vi "Builtins.vi"(6 "args":string[](array[string]), 7 "QD Plugins Dir":path, 8 "error in (no error)":errorcluster, 9 "Shift?":bool, 10 "Focus":enum8{"FP", "BD"}(ring), 11 "VI Refnum":refnum<vi>) -> (0 "error out":errorcluster)   [LabVIEW 2019]
doc: "Built-in script shortcuts\n\nUsage: Ctrl-Space + \"<shortcut>\" + Ctrl-S\n\nCreated by: Ryan Pacini\n\n[SCRIPT]\n--=Rename Label\n--c=Rename Caption\n--iconlib=Edit Library Icon\n0=Open in File Explore\na=Arrange\naa=Align Left Edges\nad=Align Right Edges\nah=Align Horizontal Centers\nas=Align Bottom Edges\nav=Align Vertical Centers\naw=Align Top Edges\nc=Connect Pane\ncf=Cluster Size Fit\nch=Cluster Size Horizontally\ncn=Cluster Size None\ncv=Cluster Size Vertically\nd=Distribute Vertical Compress\nda=Distribute Left Edges\ndd=Distribute Right Edges\ndf=Distribute Horizontal Compress \ndh=Distribute Horizontal Centers\ndhg=Distribute Horizontal Gap\nds=Distribute Bottom Edges\ndv=Distribute Vertical Centers\ndvg=Distribute Vertical Gap\ndw=Distribute Top Edges\ne=Resizes Window\ner=Error Structure\nhb=Hide Inc/Dec Buttons\nhc=Hide Caption\nhi=Hide Index Display\nhl=Hide Label\nhr=Hide Radix\nhs=Hide Scrollbars\nm=Merge Icon Layers\no=Reset Panel Origins\nrb=Radix Binary or Backslash\nrd=Radix Decimal or Normal\nrx=Radix Hex\nsb=Show Inc/Dec Buttons\nsc=Show Caption\nsi=Show Index Display\nsl=Show Label\nss=Show Scrollbars\nsel=Select Controls and Indicators\nselc=Select Controls\nseli=Select Indicators\nseln=Select None\nsg=Snap to Panel Grid\nu8=Change to U8\nu16=Change to U16\nu32=Change to U32\nu64=Change to U64\ni8=Change to I8\ni16=Change to I16\ni32=Change to I32\ni64=Change to I64\nsgl=Change to SGL\ndbl=Change to DBL\next=Change to EXT\ncsg=Change to CSG\ncdb=Change to CDB\ncxt=Change to CXT\nvi=VI Voodoo"
uses:
  _Builtins/Align.ctl
  <vilib>/numeric/LVNumericRepresentation.ctl
  _Builtins/Distribute.ctl
  _Builtins/Selection.ctl
  _Builtins/Builtins.lvlib
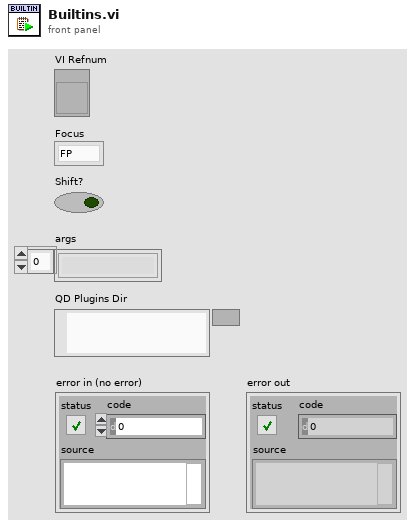
[diagram p1: front panel]
types:
  T1 = typedef "Builtins.lvlib/Align.ctl" = enum8{"Top Edges", "Vertical Centers", "Bottom Edges", "Left Edges", "Horizontal Centers", "Right Edges"}
  T2 = typedef "LVNumericRepresentation.ctl" = enum32{"Extended Precision", "Double Precision", "Single Precision", "Long", "Word", "Byte", "Unsigned Long", "Unsigned Word", "Unsigned Byte", "Complex Extended", "Complex Double", "Complex Single", "Quad", "Unsigned Quad", "Fixed-Point"}
  T3 = enum8{"None", "SizeToFit", "Horizontally", "Vertically"}
  T4 = typedef "Builtins.lvlib/Distribute.ctl" = enum8{"Top Edges", "Vertical Centers", "Bottom Edges", "Vertical Gap", "Vertical Compress", "Left Edges", "Horizontal Centers", "Right Edges", "Horizontal Gap", "Horizontal Compress"}
  T5 = typedef "Builtins.lvlib/Selection.ctl" = enum8{"None", "Controls", "Indicators", "Both"}
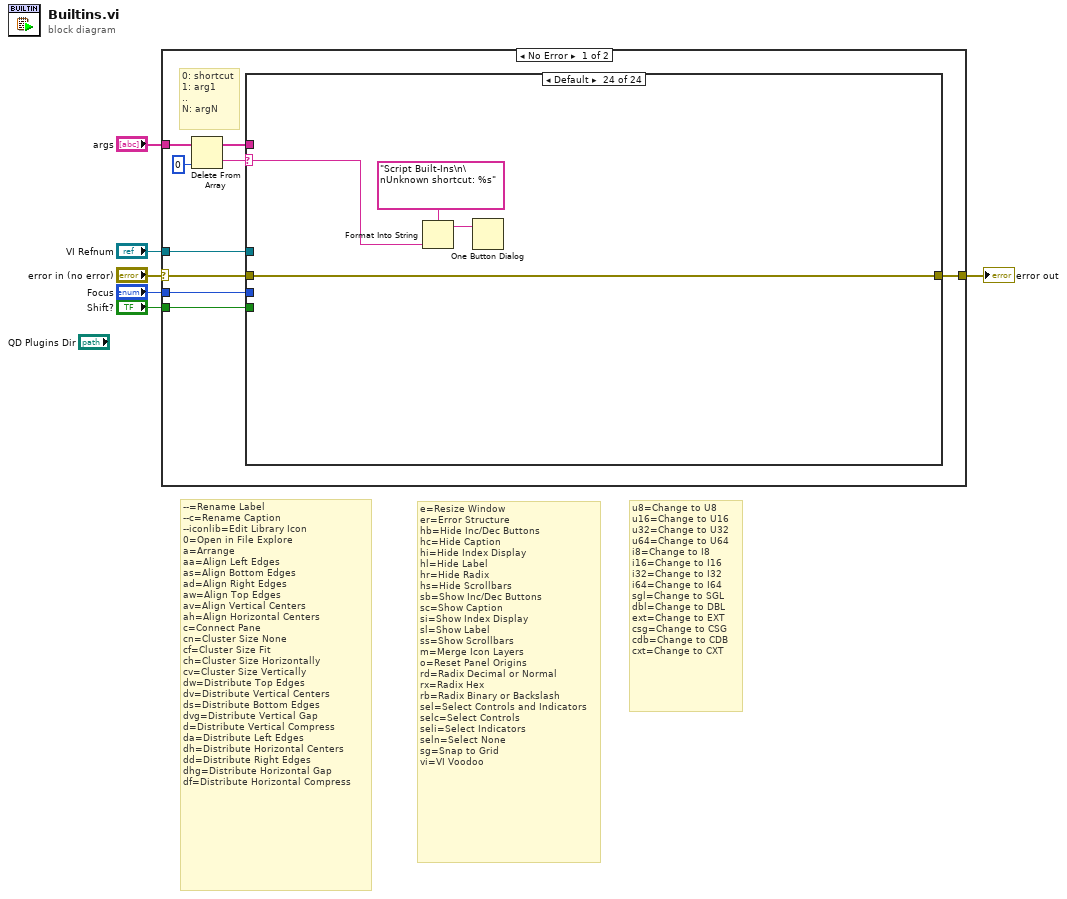
[diagram p0: block diagram]
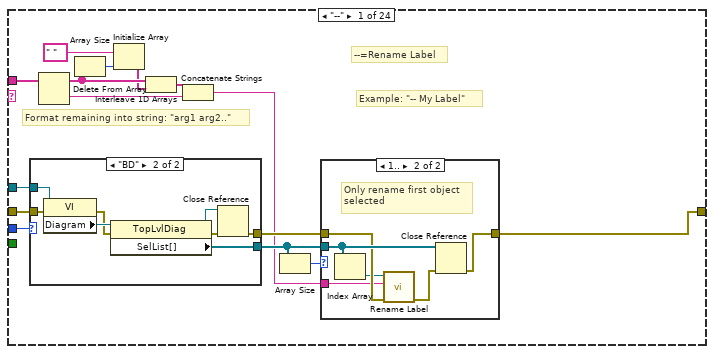
[diagram p2: hidden frame]
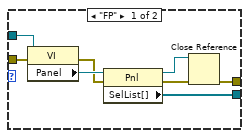
[diagram p3: hidden frame]
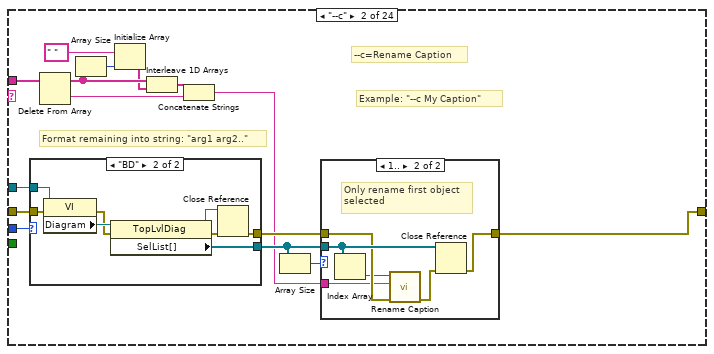
[diagram p5: hidden frame]
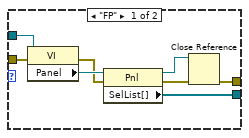
[diagram p6: hidden frame]
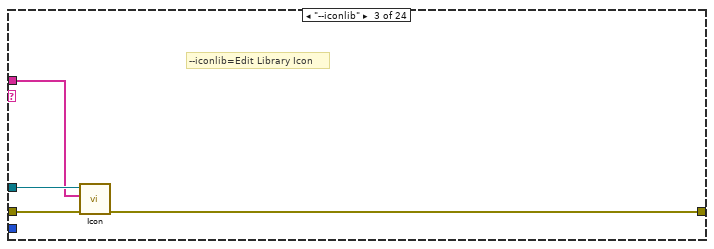
[diagram p8: hidden frame]
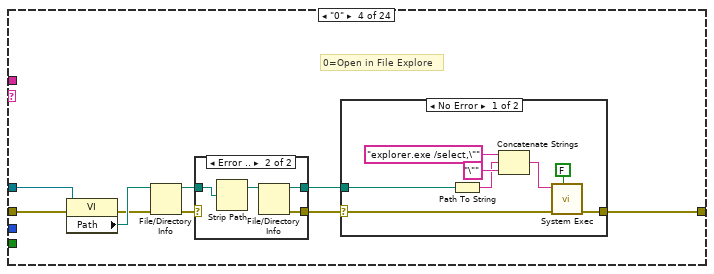
[diagram p9: hidden frame]
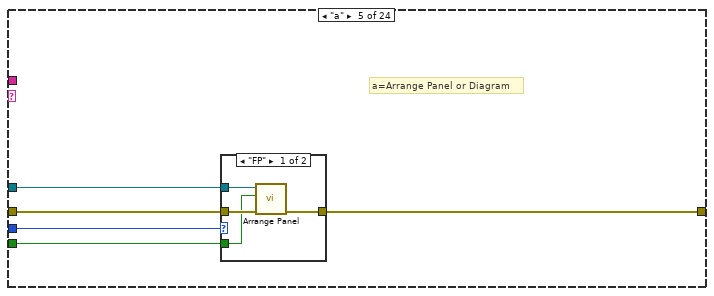
[diagram p12: hidden frame]
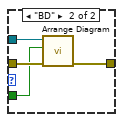
[diagram p13: hidden frame]
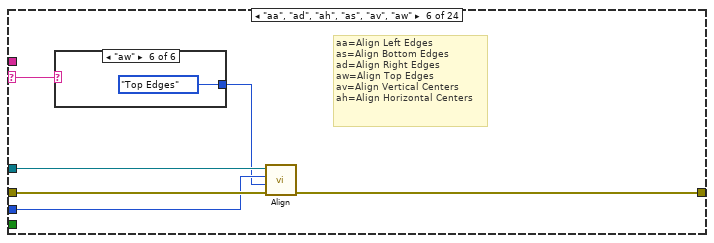
[diagram p14: hidden frame]
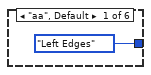
[diagram p15: hidden frame]
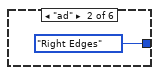
[diagram p16: hidden frame]
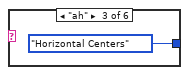
[diagram p17: hidden frame]
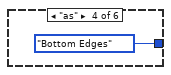
[diagram p18: hidden frame]
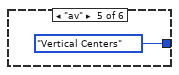
[diagram p19: hidden frame]
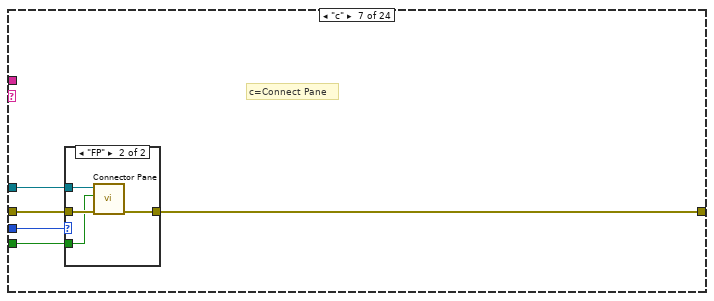
[diagram p20: hidden frame]
diagram:
  # "u8=Change to U8\nu16=Change to U16\nu32=Change to U32\nu64=Change to U64\ni8=Change to I8\ni16=Change to I16\ni32=Change to I32\ni64=Change to I64\nsgl=Change to SGL\ndbl=Change to DBL\next=Change to EXT\ncsg=Change to CSG\ncdb=Change to CDB\ncxt=Change to CXT"
  # "e=Resize Window\ner=Error Structure\nhb=Hide Inc/Dec Buttons\nhc=Hide Caption\nhi=Hide Index Display\nhl=Hide Label\nhr=Hide Radix\nhs=Hide Scrollbars\nsb=Show Inc/Dec Buttons\nsc=Show Caption\nsi=Show Index Display\nsl=Show Label\nss=Show Scrollbars\nm=Merge Icon Layers\no=Reset Panel Origins\nrd=Radix Decimal or Normal\nrx=Radix Hex\nrb=Radix Binary or Backslash\nsel=Select Controls and Indicators\nselc=Select Controls\nseli=Select Indicators\nseln=Select None\nsg=Snap to Grid\nvi=VI Voodoo"
  # "--=Rename Label\n--c=Rename Caption\n--iconlib=Edit Library Icon\n0=Open in File Explore\na=Arrange\naa=Align Left Edges\nas=Align Bottom Edges\nad=Align Right Edges\naw=Align Top Edges\nav=Align Vertical Centers\nah=Align Horizontal Centers\nc=Connect Pane\ncn=Cluster Size None\ncf=Cluster Size Fit\nch=Cluster Size Horizontally\ncv=Cluster Size Vertically\ndw=Distribute Top Edges\ndv=Distribute Vertical Centers\nds=Distribute Bottom Edges\ndvg=Distribute Vertical Gap\nd=Distribute Vertical Compress\nda=Distribute Left Edges\ndh=Distribute Horizontal Centers\ndd=Distribute Right Edges\ndhg=Distribute Horizontal Gap\ndf=Distribute Horizontal Compress"
  n1 = case shown="No Error" "error in (no error)" {
    selector: "error in (no error)" -> [w15 w387]
    tunnel: "VI Refnum" -> [w14 _]
    tunnel: "Focus" -> [w13 _]
    tunnel: "Shift?" -> [w11 _]
    tunnel: "args" -> [w10 _]
    tunnel: [w12 w387] -> w1
    frame No Error {
      # "0: shortcut\n1: arg1\n..\nN: argN"
      n2 = Delete From Array(array=w10, index=0) -> (deleted portion=w9:string, array with subset deleted=w8:string[])  [unwired: 1 in]
      n3 = case shown="Default" w9 {
        selector: w9 -> [_ _ _ _ _ w133 _ w159 w213 w223 _ _ w253 w267 w282 w296 w310 w323 _ _ w345 _ _ w385]
        tunnel: w15 -> [w30 w68 w95 w104 w124 w138 w149 w158 w212 w228 w241 w246 w252 w266 w280 w294 w308 w322 w334 w338 w349 w357 w378 w386]
        tunnel: w14 -> [w29 w67 w94 w103 w123 w137 w148 w157 w211 w227 w242 w245 w251 w265 w279 w293 w307 w321 w335 w339 w348 w356 w377 _]
        tunnel: w13 -> [w24 w62 _ _ w121 w135 w146 w155 w210 w226 w239 w243 w250 w264 w278 w292 w306 w320 _ w336 w346 w354 w372 _]
        tunnel: [w27 w65 w93 w102 w122 w136 w147 w156 w207 w225 w240 w244 w247 w261 w276 w289 w303 w317 w333 w337 w347 w355 w367 w386] -> w12
        tunnel: w11 -> [_ _ _ _ w120 _ w145 _ _ _ _ _ _ _ _ _ _ _ _ _ _ _ _ _]
        tunnel: w8 -> [w17 w55 w92 _ _ _ _ _ _ _ _ _ _ _ _ _ _ _ _ _ _ _ _ _]
        frame "--" {
          # "Example: \"-- My Label\""
          # "Format remaining into string: \"arg1 arg2..\""
          # "--=Rename Label"
          n4 = case shown="\"BD\"" w24 {
            tunnel: w30 -> [w38 w46]
            tunnel: w29 -> [w37 w45]
            tunnel: [w33 w41] -> w28
            tunnel: [w31 w39] -> w25
            frame "FP" {
              n5 = property class="VI"(reference=w37, error in=w38) -> (error out=w35:errorcluster, "Panel"=w36:refnum<vi>)  [unwired: 1 out]
              n6 = property class="Pnl"(reference=w36, error in=w35) -> (reference out=w34:refnum<vi>, error out=w32:errorcluster, "SelList[]"=w33:refnum<vi>[])
              n7 = Close Reference(reference=w34, error in (no error)=w32) -> (error out=w31:errorcluster)
            }
            frame "BD" {
              n8 = property class="VI"(reference=w45, error in=w46) -> (error out=w43:errorcluster, "Diagram"=w44:refnum<vi>)  [unwired: 1 out]
              n9 = property class="TopLvlDiag"(reference=w44, error in=w43) -> (reference out=w42:refnum<vi>, error out=w40:errorcluster, "SelList[]"=w41:refnum<vi>[])
              n10 = Close Reference(reference=w42, error in (no error)=w40) -> (error out=w39:errorcluster)
            }
          }
          n11 = Delete From Array(array=w17) -> (deleted portion=w18:string, array with subset deleted=w20:string[])  [unwired: 2 in]
          n12 = Array Size(array=w20) -> (size(s)=w22:i32)
          n13 = Initialize Array(" ", w22) -> (w19:string[])
          n14 = Interleave 1D Arrays(w20, w19) -> (w23:string[])
          n15 = Concatenate Strings(w23, w18) -> (w16:string)
          n16 = Array Size(array=w28) -> (size(s)=w26:i32)
          n17 = case shown="1.." w26 {
            tunnel: w25 -> [w47 w51]
            tunnel: w28 -> [_ w53]
            tunnel: w16 -> [_ w48]
            tunnel: [w47 w52] -> w27
            frame ..0 {
              # "Nothing selected"
            }
            frame 1.. {
              # "Only rename first object\nselected"
              n18 = Index Array(array=w53) -> (element=w50:refnum<vi>)  [unwired: 1 in]
              n19 = call "Rename Label.vi"("error in (no error)"=w51, "Label"=w48, "GObject in"=w50) -> ("error out"=w49:errorcluster)  [unwired: 6 in, 2 out]
              n20 = Close Reference(reference=w53, error in (no error)=w49) -> (error out=w52:errorcluster)
            }
          }
        }
        frame "--c" {
          # "Example: \"--c My Caption\""
          # "Format remaining into string: \"arg1 arg2..\""
          # "--c=Rename Caption"
          n21 = case shown="\"BD\"" w62 {
            tunnel: w68 -> [w76 w84]
            tunnel: w67 -> [w75 w83]
            tunnel: [w71 w79] -> w66
            tunnel: [w69 w77] -> w63
            frame "FP" {
              n22 = property class="VI"(reference=w75, error in=w76) -> (error out=w73:errorcluster, "Panel"=w74:refnum<vi>)  [unwired: 1 out]
              n23 = property class="Pnl"(reference=w74, error in=w73) -> (reference out=w72:refnum<vi>, error out=w70:errorcluster, "SelList[]"=w71:refnum<vi>[])
              n24 = Close Reference(reference=w72, error in (no error)=w70) -> (error out=w69:errorcluster)
            }
            frame "BD" {
              n25 = property class="VI"(reference=w83, error in=w84) -> (error out=w81:errorcluster, "Diagram"=w82:refnum<vi>)  [unwired: 1 out]
              n26 = property class="TopLvlDiag"(reference=w82, error in=w81) -> (reference out=w80:refnum<vi>, error out=w78:errorcluster, "SelList[]"=w79:refnum<vi>[])
              n27 = Close Reference(reference=w80, error in (no error)=w78) -> (error out=w77:errorcluster)
            }
          }
          n28 = Delete From Array(array=w55) -> (deleted portion=w56:string, array with subset deleted=w58:string[])  [unwired: 2 in]
          n29 = Array Size(array=w58) -> (size(s)=w60:i32)
          n30 = Initialize Array(" ", w60) -> (w57:string[])
          n31 = Interleave 1D Arrays(w58, w57) -> (w61:string[])
          n32 = Concatenate Strings(w61, w56) -> (w54:string)
          n33 = Array Size(array=w66) -> (size(s)=w64:i32)
          n34 = case shown="1.." w64 {
            tunnel: w63 -> [w85 w89]
            tunnel: w66 -> [_ w91]
            tunnel: w54 -> [_ w87]
            tunnel: [w85 w90] -> w65
            frame ..0 {
              # "Nothing selected"
            }
            frame 1.. {
              # "Only rename first object\nselected"
              n35 = Index Array(array=w91) -> (element=w88:refnum<vi>)  [unwired: 1 in]
              n36 = call "Rename Caption.vi"("error in (no error)"=w89, "Caption"=w87, "GObject in"=w88) -> ("error out"=w86:errorcluster)  [unwired: 6 in, 2 out]
              n37 = Close Reference(reference=w91, error in (no error)=w86) -> (error out=w90:errorcluster)
            }
          }
        }
        frame "--iconlib" {
          # "--iconlib=Edit Library Icon"
          n38 = call "Icon.vi"("error in (no error)"=w95, "Args"=w92, "VI Refnum in"=w94) -> ("error out"=w93:errorcluster)  [unwired: 7 in, 1 out]
        }
        frame "0" {
          # "0=Open in File Explore"
          n39 = property class="VI"(reference=w103, error in=w104) -> (error out=w96:errorcluster, "Path"=w101:path)  [unwired: 1 out]
          n40 = File/Directory Info(path=w101, error in=w96) -> (path out=w100:path, error out=w98:errorcluster)  [unwired: 5 out]
          n41 = case shown="Error .." w98 {
            selector: w98 -> [w105 _]
            tunnel: w100 -> [w106 w110]
            tunnel: [w105 w108] -> w99
            tunnel: [w106 w107] -> w97
            frame No Error {
            }
            frame Error {
              n42 = Strip Path(path=w110) -> (stripped path=w109:path)  [unwired: 1 out]
              n43 = File/Directory Info(path=w109) -> (path out=w107:path, error out=w108:errorcluster)  [unwired: 1 in, 5 out]
            }
          }
          n44 = case shown="No Error" w99 {
            selector: w99 -> [w111 w119]
            tunnel: [w113 w119] -> w102
            tunnel: w97 -> [w112 _]
            frame No Error {
              n45 = Path To String(path=w112) -> (string=w114:string)
              n46 = Concatenate Strings("explorer.exe /select,\"" ("string"), w114, "\"" ("string")) -> (w116:string)
              n47 = call <vilib>:"System Exec.vi"("wait until completion? (T)"=FALSE, "error in (no error)"=w111, "command line"=w116) -> ("error out"=w113:errorcluster)  [unwired: 5 in, 3 out]
            }
            frame Error {
            }
          }
        }
        frame "a" {
          # "a=Arrange Panel or Diagram"
          n48 = case shown="\"FP\"" w121 {
            tunnel: w124 -> [w128 w132]
            tunnel: w123 -> [w127 w131]
            tunnel: w120 -> [w126 w130]
            tunnel: [w125 w129] -> w122
            frame "FP" {
              n49 = call "Arrange Panel.vi"("error in (no error)"=w128, "Shift?"=w126, "VI Refnum in"=w127) -> ("error out"=w125:errorcluster)  [unwired: 7 in, 1 out]
            }
            frame "BD" {
              n50 = call "Arrange Diagram.vi"("error in (no error)"=w132, "Shift?"=w130, "VI Refnum in"=w131) -> ("error out"=w129:errorcluster)  [unwired: 7 in, 1 out]
            }
          }
        }
        frame "aa", "ad", "ah", "as", "av", "aw" {
          # "aa=Align Left Edges\nas=Align Bottom Edges\nad=Align Right Edges\naw=Align Top Edges\nav=Align Vertical Centers\nah=Align Horizontal Centers"
          n51 = case shown="\"aw\"" w133 {
            tunnel: [Align."Left Edges" ("Align Type") Align."Right Edges" ("Align Type") Align."Horizontal Centers" ("Align Type") Align."Bottom Edges" ("Align Type") Align."Vertical Centers" ("Align Type") Align."Top Edges" ("Align Type")] -> w134
            frame "aa", Default {
            }
            frame "ad" {
            }
            frame "ah" {
            }
            frame "as" {
            }
            frame "av" {
            }
            frame "aw" {
            }
          }
          n52 = call "Align.vi"("error in (no error)"=w138, "Align Type"=w134, "Panel"=w135, "VI Refnum in"=w137) -> ("error out"=w136:errorcluster)  [unwired: 6 in, 1 out]
        }
        frame "c" {
          # "c=Connect Pane"
          n53 = case shown="\"FP\"" w146 {
            tunnel: w149 -> [w150 w154]
            tunnel: w148 -> [_ w153]
            tunnel: [w150 w152] -> w147
            tunnel: w145 -> [_ w151]
            frame "BD" {
            }
            frame "FP" {
              n54 = call "Connector Pane.vi"("error in (no error)"=w154, "Wire Middle? (F)"=w151, "VI Refnum in"=w153) -> ("error out"=w152:errorcluster)  [unwired: 7 in, 1 out]
            }
          }
        }
        frame "cdb", "csg", "cxt", "dbl", "ext", "i16", "i32", "i64", "i8", "sgl", "u16", "u32", "u64", "u8" {
          # "**WARNING: Changing Representation clears the panel/diagram Selection List (LV2019 bug)"
          # "sgl=Change to SGL\ndbl=Change to DBL\next=Change to EXT\ncsg=Change to CSG\ncdb=Change to CDB\ncxt=Change to CXT"
          # "u8=Change to U8\nu16=Change to U16\nu32=Change to U32\nu64=Change to U64\ni8=Change to I8\ni16=Change to I16\ni32=Change to I32\ni64=Change to I64"
          n55 = case shown="\"u8\", Default" w159 {
            tunnel: [LVNumericRepresentation."Unsigned Byte" ("Representation") LVNumericRepresentation."Unsigned Word" ("Representation") LVNumericRepresentation."Unsigned Long" ("Representation") LVNumericRepresentation."Unsigned Quad" ("Representation") LVNumericRepresentation."Byte" ("Representation") LVNumericRepresentation."Word" ("Representation") LVNumericRepresentation."Long" ("Representation") LVNumericRepresentation."Quad" ("Representation") LVNumericRepresentation."Single Precision" ("Representation") LVNumericRepresentation."Double Precision" ("Representation") LVNumericRepresentation."Extended Precision" ("Representation") LVNumericRepresentation."Complex Single" ("Representation") LVNumericRepresentation."Complex Double" ("Representation") LVNumericRepresentation."Complex Extended" ("Representation")] -> w160
            frame "u8", Default {
            }
            frame "u16" {
            }
            frame "u32" {
            }
            frame "u64" {
            }
            frame "i8" {
            }
            frame "i16" {
            }
            frame "i32" {
            }
            frame "i64" {
            }
            frame "sgl" {
            }
            frame "dbl" {
            }
            frame "ext" {
            }
            frame "csg" {
            }
            frame "cdb" {
            }
            frame "cxt" {
            }
          }
          n56 = case shown="\"FP\"" w155 {
            tunnel: w160 -> [w172 w188]
            tunnel: w158 -> [w169 w185]
            tunnel: w157 -> [w168 w184]
            tunnel: [w162 w178] -> w156
            frame "BD" {
              n57 = property class="VI"(reference=w168, error in=w169) -> (error out=w170:errorcluster, "Diagram"=w171:refnum<vi>)  [unwired: 1 out]
              n58 = property class="TopLvlDiag"(reference=w171, error in=w170) -> (reference out=w166:refnum<vi>, error out=w167:errorcluster, "SelList[]"=w165:refnum<vi>[])
              n59 = for {
                tunnel: w165 -> [w176] mode=indexing
                tunnel: w172 -> [w175]
                shift-right: [w173] -> w164
                shift-left: w167 -> [w174]
                n60 = call "Numeric Representation.vi"("error in (no error)"=w174, "Representation"=w175, "GObject in"=w176) -> ("error out"=w173:errorcluster)  [unwired: 6 in, 2 out]
              }
              n61 = invoke class="TopLvlDiag" method="Make Selection"(reference=w166, error in=w164, "Objects"=w165) -> (reference out=w161:refnum<vi>, error out=w163:errorcluster)  [unwired: 1 in, 2 out]
              n62 = Close Reference(reference=w161, error in (no error)=w163) -> (error out=w162:errorcluster)
            }
            frame "FP" {
              n63 = property class="VI"(reference=w184, error in=w185) -> (error out=w186:errorcluster, "Panel"=w187:refnum<vi>)  [unwired: 1 out]
              n64 = property class="Pnl"(reference=w187, error in=w186) -> (reference out=w182:refnum<vi>, error out=w183:errorcluster, "SelList[]"=w181:refnum<vi>[])
              n65 = for {
                tunnel: w181 -> [w192] mode=indexing
                tunnel: w188 -> [w191]
                shift-right: [w189] -> w180
                shift-left: w183 -> [w190]
                n66 = call "Numeric Representation.vi"("error in (no error)"=w190, "Representation"=w191, "GObject in"=w192) -> ("error out"=w189:errorcluster)  [unwired: 6 in, 2 out]
              }
              n67 = invoke class="Pnl" method="Make Selection"(reference=w182, error in=w180, "Objects"=w181) -> (reference out=w177:refnum<vi>, error out=w179:errorcluster)  [unwired: 1 in, 2 out]
              n68 = Close Reference(reference=w177, error in (no error)=w179) -> (error out=w178:errorcluster)
            }
          }
        }
        frame "cf", "ch", "cn", "cv" {
          # "cn=Cluster Size None\ncf=Cluster Size Fit\nch=Cluster Size Horizontally\ncv=Cluster Size Vertically"
          n69 = case shown="\"cf\"" w213 {
            tunnel: [T3."SizeToFit" ("AutoSize") T3."Horizontally" ("AutoSize") T3."None" ("AutoSize") T3."Vertically" ("AutoSize")] -> w214
            frame "cf" {
            }
            frame "ch" {
            }
            frame "cn" {
            }
            frame "cv", Default {
            }
          }
          n70 = call "Selection List.vi"("error in (no error)"=w212, "Focus"=w210, "VI Refnum in"=w211) -> ("error out"=w209:errorcluster, "SelList[]"=w208:refnum<vi>[])  [unwired: 5 in, 2 out]
          n71 = for {
            tunnel: w208 -> [w216] mode=indexing
            tunnel: w214 -> [w215]
            shift-right: [w217] -> w207
            shift-left: w209 -> [w218]
            n72 = call "Cluster Autosize.vi"("error in (no error)"=w218, "AutoSize"=w215, "GObject in"=w216) -> ("error out"=w217:errorcluster)  [unwired: 6 in, 2 out]
          }
        }
        frame "d", "da", "dd", "df", "dh", "dhg", "ds", "dv", "dvg", "dw" {
          # "dw=Distribute Top Edges\ndv=Distribute Vertical Centers\nds=Distribute Bottom Edges\ndvg=Distribute Vertical Gap\nd=Distribute Vertical Compress\nda=Distribute Left Edges\ndh=Distribute Horizontal Centers\ndd=Distribute Right Edges\ndhg=Distribute Horizontal Gap\ndf=Distribute Horizontal Compress"
          n73 = case shown="\"d\", Default" w223 {
            tunnel: [Distribute."Vertical Compress" ("Distribute Type") Distribute."Left Edges" ("Distribute Type") Distribute."Right Edges" ("Distribute Type") Distribute."Horizontal Compress" ("Distribute Type") Distribute."Horizontal Centers" ("Distribute Type") Distribute."Horizontal Gap" ("Distribute Type") Distribute."Bottom Edges" ("Distribute Type") Distribute."Vertical Centers" ("Distribute Type") Distribute."Vertical Gap" ("Distribute Type") Distribute."Top Edges" ("Distribute Type")] -> w224
            frame "d", Default {
            }
            frame "da" {
            }
            frame "dd" {
            }
            frame "df" {
            }
            frame "dh" {
            }
            frame "dhg" {
            }
            frame "ds" {
            }
            frame "dv" {
            }
            frame "dvg" {
            }
            frame "dw" {
            }
          }
          n74 = call "Distribute.vi"("error in (no error)"=w228, "Distribute Type"=w224, "Panel"=w226, "VI Refnum in"=w227) -> ("error out"=w225:errorcluster)  [unwired: 6 in, 1 out]
        }
        frame "e" {
          # "e=Resize Window"
          n75 = call "Resize Window.vi"("error in (no error)"=w241, "Focus"=w239, "VI Refnum in"=w242) -> ("error out"=w240:errorcluster)  [unwired: 7 in, 1 out]
        }
        frame "er" {
          # "er=Error Structure"
          n76 = call "Error Structure.vi"("error in (no error)"=w246, "Focus"=w243, "VI Refnum in"=w245) -> ("error out"=w244:errorcluster)  [unwired: 7 in, 1 out]
        }
        frame "hb", "sb" {
          # "hb=Hide Inc/Dec Buttons\nsb=Show Inc/Dec Buttons"
          n77 = case shown="\"sb\"" w253 {
            tunnel: [enum8{"hide", "show"}."hide" ("inc/dec") enum8{"hide", "show"}."show" ("inc/dec")] -> w254
            frame "hb", Default {
            }
            frame "sb" {
            }
          }
          n78 = call "Selection List.vi"("error in (no error)"=w252, "Focus"=w250, "VI Refnum in"=w251) -> ("error out"=w249:errorcluster, "SelList[]"=w248:refnum<vi>[])  [unwired: 5 in, 2 out]
          n79 = for {
            tunnel: w248 -> [w258] mode=indexing
            tunnel: w254 -> [w255]
            shift-right: [w256] -> w247
            shift-left: w249 -> [w257]
            n80 = call "Visible IncDec.vi"("error in (no error)"=w257, "inc/dec"=w255, "GObject in"=w258) -> ("error out"=w256:errorcluster)  [unwired: 5 in, 3 out]
          }
        }
        frame "hs", "ss" {
          # "hs=Hide Scrollbars\nss=Show Scrollbars"
          n81 = case shown="\"hs\", Default" w267 {
            tunnel: [enum8{"hide", "show"}."hide" ("inc/dec") enum8{"hide", "show"}."show" ("inc/dec")] -> w268
            frame "hs", Default {
            }
            frame "ss" {
            }
          }
          n82 = call "Selection List.vi"("error in (no error)"=w266, "Focus"=w264, "VI Refnum in"=w265) -> ("error out"=w263:errorcluster, "SelList[]"=w262:refnum<vi>[])  [unwired: 5 in, 2 out]
          n83 = for {
            tunnel: w262 -> [w270] mode=indexing
            tunnel: w268 -> [w269]
            shift-right: [w271] -> w261
            shift-left: w263 -> [w272]
            n84 = call "Visible Scrollbar.vi"("error in (no error)"=w272, "scrollbars"=w269, "GObject in"=w270) -> ("error out"=w271:errorcluster)  [unwired: 5 in, 3 out]
          }
        }
        frame "hc", "sc" {
          # "hc=Hide Caption\nsc=Show Caption"
          n85 = case shown="\"sc\", Default" w282 {
            tunnel: [enum8{"hide", "show"}."hide" ("label") enum8{"hide", "show"}."show" ("label")] -> w281
            frame "hc" {
            }
            frame "sc", Default {
            }
          }
          n86 = call "Selection List.vi"("error in (no error)"=w280, "Focus"=w278, "VI Refnum in"=w279) -> ("error out"=w277:errorcluster, "SelList[]"=w275:refnum<vi>[])  [unwired: 5 in, 2 out]
          n87 = for {
            tunnel: w275 -> [w286] mode=indexing
            shift-right: [w285] -> w276
            shift-left: w277 -> [w284]
            tunnel: w281 -> [w283]
            n88 = call "Visible Caption.vi"("error in (no error)"=w284, "caption"=w283, "GObject in"=w286) -> ("error out"=w285:errorcluster)  [unwired: 5 in, 3 out]
          }
        }
        frame "hi", "si" {
          # "hi=Hide Index Display\nsi=Show Index Display"
          n89 = case shown="\"si\", Default" w296 {
            tunnel: [enum8{"hide", "show"}."hide" ("label") enum8{"hide", "show"}."show" ("label")] -> w295
            frame "hi" {
            }
            frame "si", Default {
            }
          }
          n90 = call "Selection List.vi"("error in (no error)"=w294, "Focus"=w292, "VI Refnum in"=w293) -> ("error out"=w291:errorcluster, "SelList[]"=w290:refnum<vi>[])  [unwired: 5 in, 2 out]
          n91 = for {
            tunnel: w290 -> [w300] mode=indexing
            shift-right: [w297] -> w289
            shift-left: w291 -> [w298]
            tunnel: w295 -> [w299]
            n92 = call "Visible Index.vi"("error in (no error)"=w298, "index display"=w299, "GObject in"=w300) -> ("error out"=w297:errorcluster)  [unwired: 5 in, 3 out]
          }
        }
        frame "hl", "sl" {
          # "hl=Hide Label\nsl=Show Label"
          n93 = case shown="\"hl\"" w310 {
            tunnel: [enum8{"hide", "show"}."hide" ("label") enum8{"hide", "show"}."show" ("label")] -> w309
            frame "hl" {
            }
            frame "sl", Default {
            }
          }
          n94 = call "Selection List.vi"("error in (no error)"=w308, "Focus"=w306, "VI Refnum in"=w307) -> ("error out"=w305:errorcluster, "SelList[]"=w304:refnum<vi>[])  [unwired: 5 in, 2 out]
          n95 = for {
            tunnel: w304 -> [w314] mode=indexing
            shift-right: [w313] -> w303
            shift-left: w305 -> [w312]
            tunnel: w309 -> [w311]
            n96 = call "Visible Label.vi"("error in (no error)"=w312, "label"=w311, "GObject in"=w314) -> ("error out"=w313:errorcluster)  [unwired: 5 in, 3 out]
          }
        }
        frame "hr", "rb", "rd", "rx" {
          # "hr=Radix Hide\nrd=Radix Decimal or Normal\nrx=Radix Hex\nrb=Radix Binary or Backslash"
          n97 = case shown="\"hr\"" w323 {
            tunnel: [enum8{"hide", "dec", "hex", "bin"}."hide" ("radix") enum8{"hide", "dec", "hex", "bin"}."dec" ("radix") enum8{"hide", "dec", "hex", "bin"}."hex" ("radix") enum8{"hide", "dec", "hex", "bin"}."bin" ("radix")] -> w324
            frame "hr" {
            }
            frame "rd", Default {
            }
            frame "rx" {
            }
            frame "rb" {
            }
          }
          n98 = call "Selection List.vi"("error in (no error)"=w322, "Focus"=w320, "VI Refnum in"=w321) -> ("error out"=w319:errorcluster, "SelList[]"=w318:refnum<vi>[])  [unwired: 5 in, 2 out]
          n99 = for {
            tunnel: w318 -> [w328] mode=indexing
            tunnel: w324 -> [w326]
            shift-right: [w325] -> w317
            shift-left: w319 -> [w327]
            n100 = call "Radix.vi"("error in (no error)"=w327, "radix"=w326, "GObject in"=w328) -> ("error out"=w325:errorcluster)  [unwired: 6 in, 2 out]
          }
        }
        frame "m" {
          # "m=Merge Icon Layers"
          n101 = call "Icon Merge Layers.vi"("error in (no error)"=w334, "VI Refnum in"=w335) -> ("error out"=w333:errorcluster)  [unwired: 8 in, 1 out]
        }
        frame "o" {
          # "o=Reset Panel Origins"
          n102 = case shown="\"FP\"" w336 {
            tunnel: w339 -> [_ w343]
            tunnel: w338 -> [w340 w342]
            tunnel: [w340 w341] -> w337
            frame "BD" {
            }
            frame "FP" {
              n103 = call "Reset Origins.vi"("error in (no error)"=w342, "VI Refnum in"=w343) -> ("error out"=w341:errorcluster)  [unwired: 8 in, 1 out]
            }
          }
        }
        frame "sel", "selc", "seli", "seln" {
          # "sel=Select Controls and Indicators\nselc=Select Controls\nseli=Select Indicators\nseln=Select None"
          n104 = case shown="\"seln\", Default" w345 {
            tunnel: [Selection."Controls" ("Selection") Selection."None" ("Selection") Selection."Indicators" ("Selection") Selection."Both" ("Selection")] -> w344
            frame "selc" {
            }
            frame "seln", Default {
            }
            frame "seli" {
            }
            frame "sel" {
            }
          }
          n105 = call "Select Controls.vi"("error in (no error)"=w349, "Selection"=w344, "Focus"=w346, "VI Refnum in"=w348) -> ("error out"=w347:errorcluster)  [unwired: 6 in, 1 out]
        }
        frame "sg" {
          # "sg=Snap to Grid"
          n106 = case shown="\"FP\"" w354 {
            tunnel: w357 -> [w358 w359]
            tunnel: w356 -> [_ w360]
            tunnel: [w358 w361] -> w355
            frame "BD" {
            }
            frame "FP" {
              n107 = call "Snap to Grid.vi"("error in (no error)"=w359, "VI Refnum in"=w360) -> ("error out"=w361:errorcluster)  [unwired: 8 in, 1 out]
            }
          }
        }
        frame "vi" {
          # "1. Select all controls\n2. Hide inc/dec buttons\n3. Snap to grid with offset\n4. Reset Panel Origins\n5. Connect pane"
          # "vi=VI Voodoo"
          n108 = call "Select Controls.vi"("error in (no error)"=w378, "Selection"=Selection."Both", "Focus"=w372, "VI Refnum in"=w377) -> ("error out"=w375:errorcluster, "VI Refnum out"=w373:refnum<vi>)  [unwired: 6 in]
          n109 = call "Selection List.vi"("error in (no error)"=w375, "Focus"=w372, "VI Refnum in"=w373) -> ("error out"=w374:errorcluster, "SelList[]"=w371:refnum<vi>[], "VI Refnum out"=w368:refnum<vi>)  [unwired: 5 in, 1 out]
          n110 = for {
            tunnel: w371 -> [w381] mode=indexing
            shift-right: [w380] -> w369
            shift-left: w374 -> [w382]
            tunnel: enum8{"hide", "show"}."hide" ("label") -> [w379]
            n111 = call "Visible IncDec.vi"("error in (no error)"=w382, "inc/dec"=w379, "GObject in"=w381) -> ("error out"=w380:errorcluster)  [unwired: 5 in, 3 out]
          }
          n112 = call "Snap to Grid.vi"("error in (no error)"=w369, "VI Refnum in"=w368) -> ("error out"=w366:errorcluster, "VI Refnum out"=w364:refnum<vi>)  [unwired: 8 in]
          n113 = call "Reset Origins.vi"("error in (no error)"=w366, "VI Refnum in"=w364) -> ("error out"=w365:errorcluster, "VI Refnum out"=w363:refnum<vi>)  [unwired: 8 in]
          n114 = call "Connector Pane.vi"("error in (no error)"=w365, "Wire Middle? (F)"=FALSE, "VI Refnum in"=w363) -> ("error out"=w367:errorcluster)  [unwired: 7 in, 1 out]
        }
        frame Default {
          n115 = Format Into String(format string="Script Built-Ins\n\nUnknown shortcut: %s", w385) -> (resulting string=w383:string)  [unwired: 2 in, 1 out]
          n116 = One Button Dialog(message=w383) -> ()  [unwired: 1 in, 1 out]
        }
      }
    }
    frame Error {
    }
  }
  "error out" <- w1
